vi "SolveIKPosition.vi"(4 "error in":errorcluster, 5 "Pose":T2={"Position"={"x"=0.457, "y"=-0.385, "z"=-0.261}, "Orientation"={"Roll (y)"=3.13, "Pitch (x)"=-0.1, "Yaw (z)"=-1.85}}, 6 "Side":T3, 7 "node":string) -> (0 "error out":errorcluster)   [LabVIEW 2010]
uses:
  <userlib>/ROSforLV_0.1/ROS/Code/SubVIs/BaxterSide.ctl
  <userlib>/ROSforLV_0.1/ROS/MessageBuilding/Primitives/subs/u32Scalar.vi
panel:
  out "IK Reply":T1
  out "Reply":string
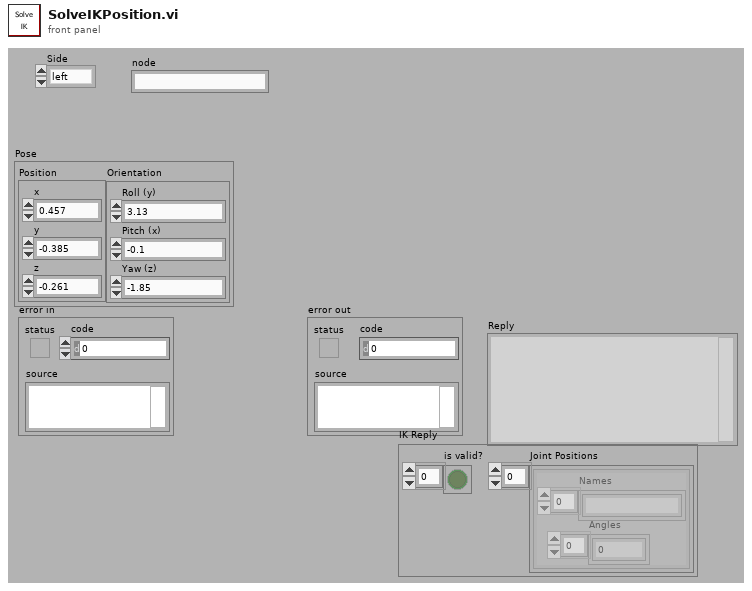
[diagram p1: front panel]
types:
  T1 = cluster{"is valid?":bool[], "Joint Positions":cluster{"Angles":dbl[], "Names":string[]}[]}
  T2 = cluster{"Position":cluster{"x":dbl, "y":dbl, "z":dbl}, "Orientation":cluster{"Roll (y)":dbl, "Pitch (x)":dbl, "Yaw (z)":dbl}}
  T3 = typedef "BaxterSide.ctl" = enum16{"left", "right"}
  T4 = cluster{"Roll (y)":dbl, "Pitch (x)":dbl, "Yaw (z)":dbl}
  T5 = typedef "_ROSControl.ctl" = cluster{"topic port":u16, "Node":string, "topic":string, "type":string, "node port":u32, "error ":errorcluster, "Direction":T6, "APIs":string[]}
  T6 = typedef "_ROSDirection.ctl" = enum16{"Node", "Publisher", "Subscriber", "Service Client"}
  T7 = cluster{"Position":cluster{"x":dbl, "y":dbl, "z":dbl}, "Quaternion":cluster{"x":dbl, "y":dbl, "z":dbl, "w":dbl}}
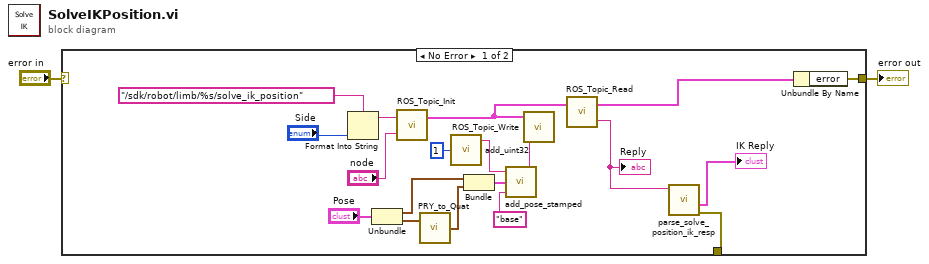
[diagram p0: block diagram]
diagram:
  n1 = case shown="No Error" "error in" {
    selector: "error in" -> [_ w22]
    tunnel: [w21 w22] -> w2
    tunnel: [w4 _] -> _
    frame No Error {
      n2 = Format Into String(format string="/sdk/robot/limb/%s/solve_ik_position" ("topic"), "Side") -> (resulting string=w18:string)  [unwired: 2 in, 1 out]
      n3 = Unbundle("Pose") -> ("Position"=w13:cluster{"x":dbl, "y":dbl, "z":dbl}, "Orientation"=w15:T4)
      n4 = call <userlib>:"ROS_Topic_Init.vi"("node"="node", "topic"=w18) -> ("ROS out"=w7:T5)  [unwired: 1 in]
      n5 = call <userlib>:"PRY_to_Quat.vi"("Orientation"=w15) -> ("Quaternion"=w14:cluster{"x":dbl, "y":dbl, "z":dbl, "w":dbl})  [unwired: 1 in]
      n6 = call-poly <userlib>:"add_uint32.vi"("Numeric"=u32 1) -> ("msg out"=w8:string)  [unwired: 4 in]
      n7 = Bundle("Position"=w13, "Quaternion"=w14) -> (w12:T7)  [unwired: 1 in]
      n8 = call <userlib>:"add_pose_stamped.vi"("frame_id"="base", "Pose"=w12, "msg in"=w8) -> ("msg out"=w9:string)  [unwired: 2 in]
      n9 = call <userlib>:"ROS_Topic_Write.vi"("Msg in"=w9, "ROS in"=w7) -> ()  [unwired: 2 in, 1 out]
      n10 = call <userlib>:"ROS_Topic_Read.vi"("ROS in"=w7) -> ("Reply"=w5:string, "ROS out"=w17:T5)  [unwired: 1 in]
      "Reply" <- w5
      n11 = call <userlib>:"parse_solve_position_ik_resp.vi"("msg in"=w5) -> ("error out"=w4:errorcluster, "IK Reply"=→"IK Reply":T1)  [unwired: 3 in, 2 out]
      n12 = Unbundle By Name(w17) -> ("error"=w21:errorcluster)
    }
    frame Error {
    }
  }
  "error out" <- w2
